vi "总磷氨氮测量流程.vi"(10 "总磷量程模式":T1, 11 "参数":T2={"站号"=1, "量程切换"=enum."AUTO", "控制命令"=enum."启动测量", "模式设置"=enum."待机", "测量间隔"=0} {"站号" items=["总磷"=1, "总氮"=2]}) -> ()   [LabVIEW 2016, in "斯坦道仪器.lvlib"]
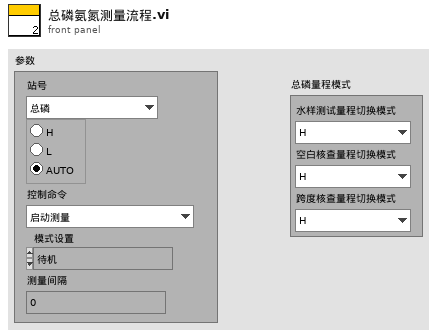
[diagram p1: front panel]
types:
  T1 = cluster{"水样测试量程切换模式":enum16{"H", "L", "AUTO"}, "空白核查量程切换模式":enum16{"H", "L", "AUTO"}, "跨度核查量程切换模式":enum16{"H", "L", "AUTO"}}
  T2 = cluster{"站号":u16, "量程切换":enum32{"H", "L", "AUTO"}, "控制命令":enum16{"启动测量", "标样核查", "零点核查", "跨度核查", "空白测试", "平行样测试", "加标回收", "空白校准", "标样校准", "初始化（清洗）", "停止测试", "仪器重启", "校时", "模式设置", "测量间隔设置"}, "模式设置":enum16{"待机", "连续模式", "周期模式", "定点模式", "受控模式", "手动模式"}, "测量间隔":u16}
  T3 = enum16{"初始化", "通电", "参数1启动", "等待参数1测试完成", "参数1测试完成", "参数1存储数据", "参数2启动", "等待参数2测试完成", "参数2测试完成", "参数2存储数据", "断电", "结束"}
  T4 = cluster{"时间标识":timestamp, "设备":string, "日志信息":string, "流程参数":string}
  T5 = cluster{"时间标识":timestamp, "监测值":sgl, "单位":u16, "数据标识":string, "因子编码":u32, "标样参考值":sgl, "F0":sgl, "F1":sgl, "F2":sgl, "F3":sgl, "F4":sgl, "F5":sgl, "F6":sgl, "F7":sgl, "X":sgl, "温度":sgl, "湿度":sgl, "量程标识":string}
  T6 = enum16{"维护数据", "水样测试", "标样核查", "零点核查", "跨度核查", "空白测试", "平行样测试", "加标回收", "空白校准", "标样校准", "初始化（清洗）"}
  T7 = enum16{"启动测量", "标样核查", "零点核查", "跨度核查", "空白测试", "平行样测试", "加标回收", "空白校准", "标样校准", "初始化（清洗）", "停止测试", "仪器重启", "校时", "模式设置", "测量间隔设置"}
  T8 = cluster{"系统时间":timestamp, "工作状态":enum16{"空闲", "水样测试", "标样核查", "零点核查", "跨度核查", "空白测试", "平行样测试", "加标回收", "空白校准", "标样校准", "初始化（清洗）"}, "测量模式":enum16{"待机", "连续模式", "周期模式", "定点模式", "受控模式", "手动模式"}, "告警代码":enum16{"无告警", "缺试剂告警", "缺水样告警", "缺蒸馏水告警", "缺标液告警", "仪表漏液告警", "标定异常告警", "超量程告警", "加热异常", "低试剂预警", "超上限告警", "超下限告警", "仪表内部其他异常", "滴定异常告警", "电极异常告警", "量程切换告警", "参数设置告警", "PH电极电位异常", "电导率电极异常", "浊度光度异常", "溶解氧电极异常", "溶解氧光强异常", "温度异常告警", "PH异常告警", "溶解氧异常告警", "电导率异常告警", "浊度异常告警", "叶绿素异常告警", "藻密度异常告警", "蓝绿藻异常告警", "ORP异常告警", "氨氮异常告警", "清洁刷异常告警", "SD卡异常告警", "蓝牙异常告警", "Wifi异常告警", "流程异常告警"}, "故障代码":enum16{"无故障", "电机故障", "温度故障", "通讯故障", "滴定故障"}, "日志代码":u16, "软件版本":u16, "F0":sgl, "F1":sgl, "F2":sgl, "F3":sgl, "T":sgl, "H":sgl, "id":u16, "flowid":u16, "量程":u16, "总磷控温温度1":sgl, "营养盐控温温度2":sgl, "ADC":sgl}
  T9 = enum16{"空闲", "水样测试", "标样核查", "零点核查", "跨度核查", "空白测试", "平行样测试", "加标回收", "空白校准", "标样校准", "初始化（清洗）"}
  T10 = cluster{"因子编码":u32, "单位":u16, "标样参考值":sgl, "水样数据时间":timestamp, "水样实测值":sgl, "水样数据标识":string, "标样数据时间":timestamp, "标样实测值":sgl, "标样数据标识":string, "空白数据时间":timestamp, "空白实测值":sgl, "空白数据标识":string, "零点核查数据时间":timestamp, "零点核查实测值":sgl, "零点核查数据标识":string, "跨度核查数据时间":timestamp, "跨度核查实测值":sgl, "跨度核查数据标识":string, "加标回收数据时间":timestamp, "加标回收实测值":sgl, "加标回收数据标识":string, "平行样数据时间":timestamp, "平行样实测值":sgl, "平行样数据标识":string, "F0":sgl, "F1":sgl, "F2":sgl, "F3":sgl, "F4":sgl, "F5":sgl, "F6":sgl, "F7":sgl, "温度":sgl, "湿度":sgl, "X值":sgl}
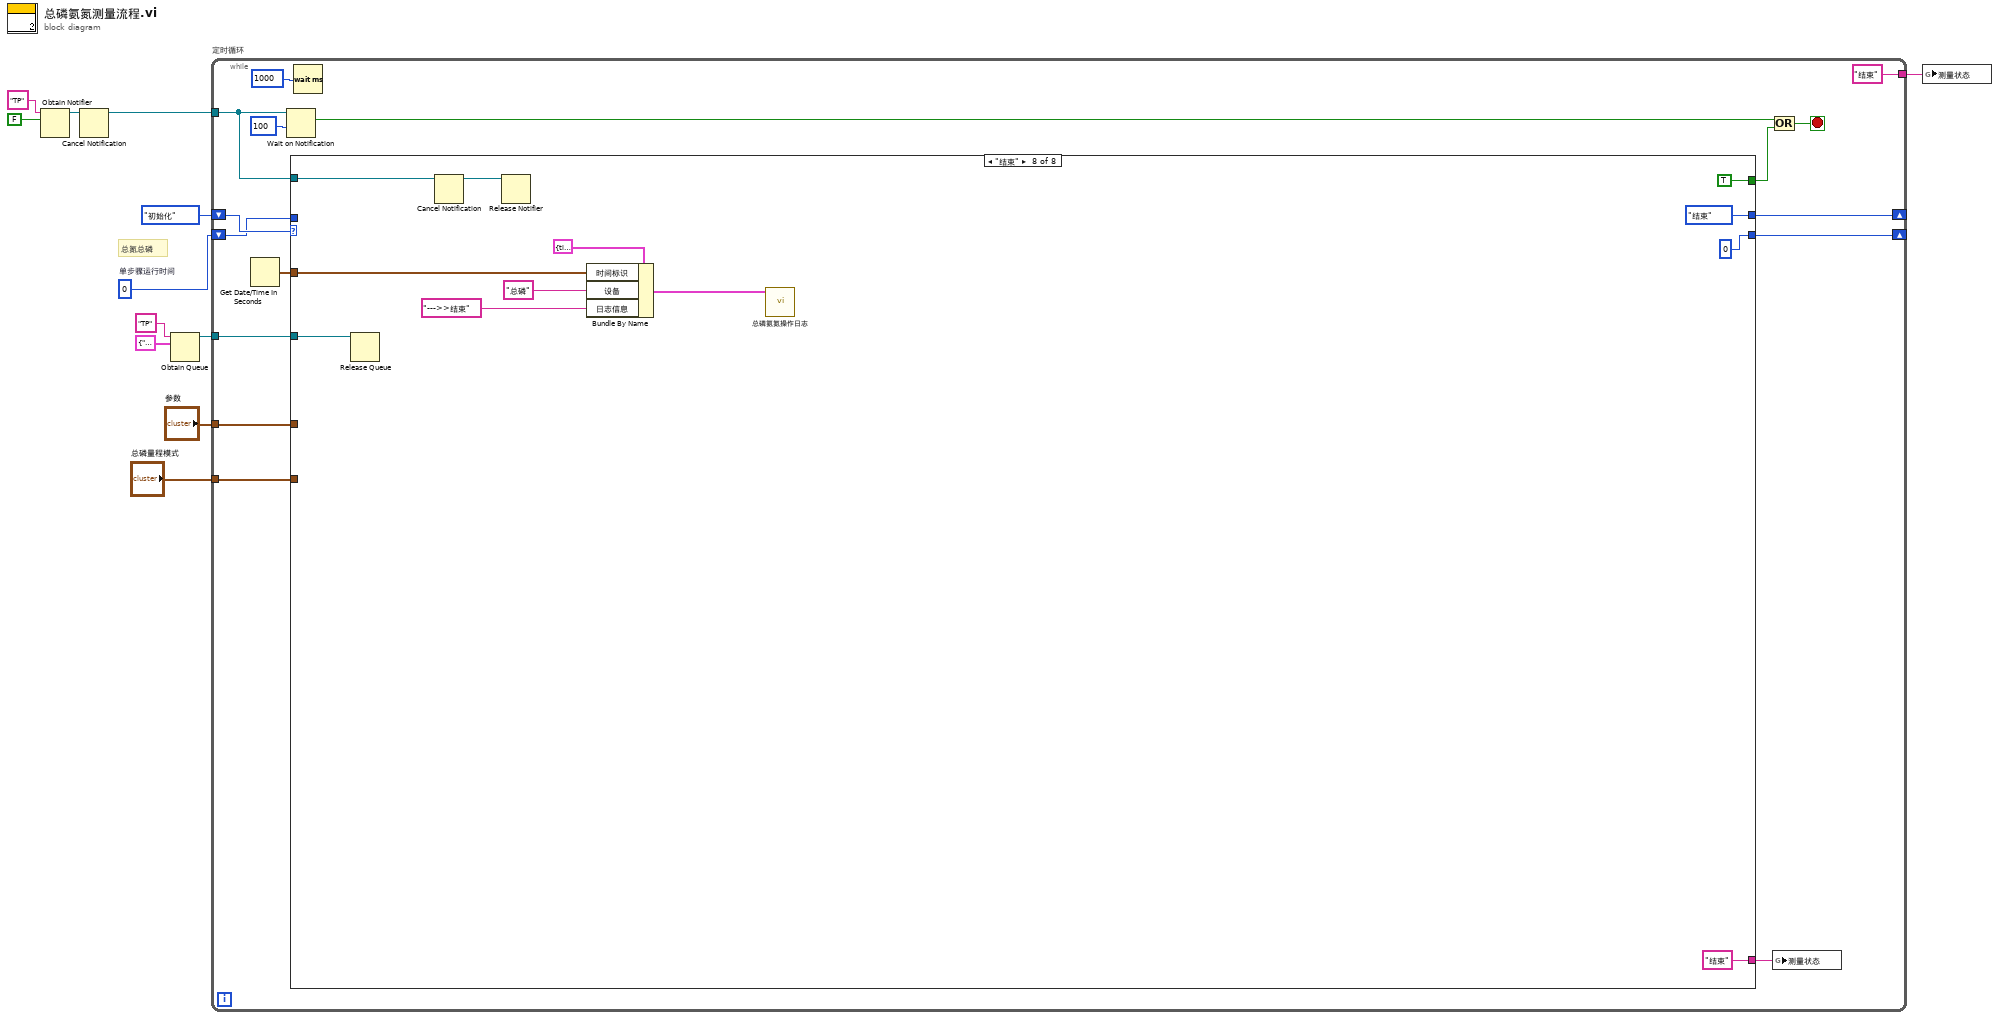
[diagram p0: block diagram]
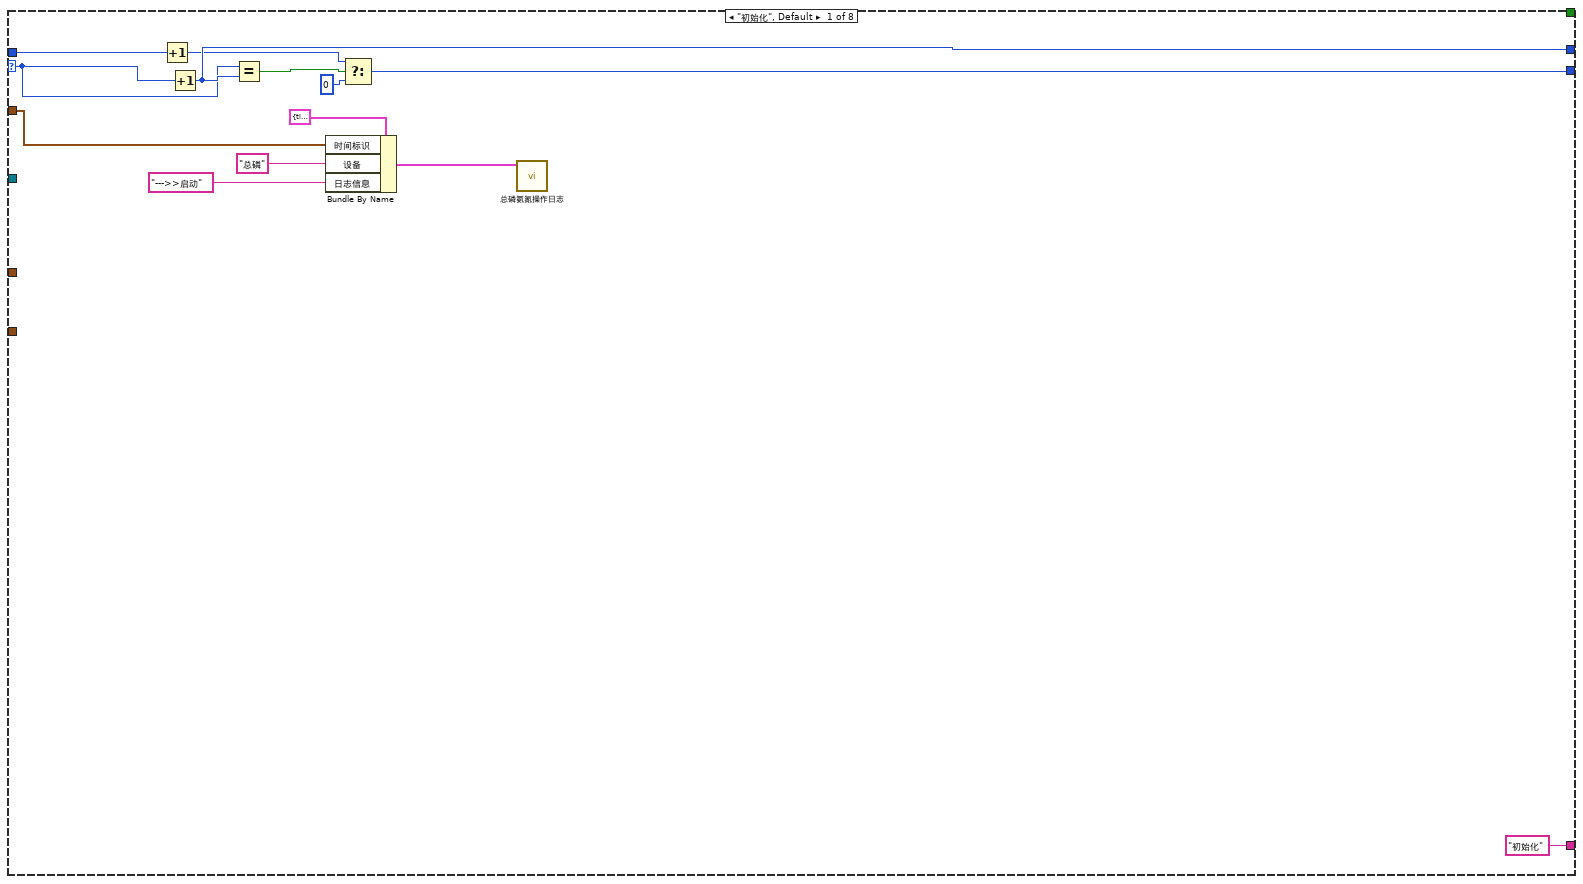
[diagram p2: hidden frame]
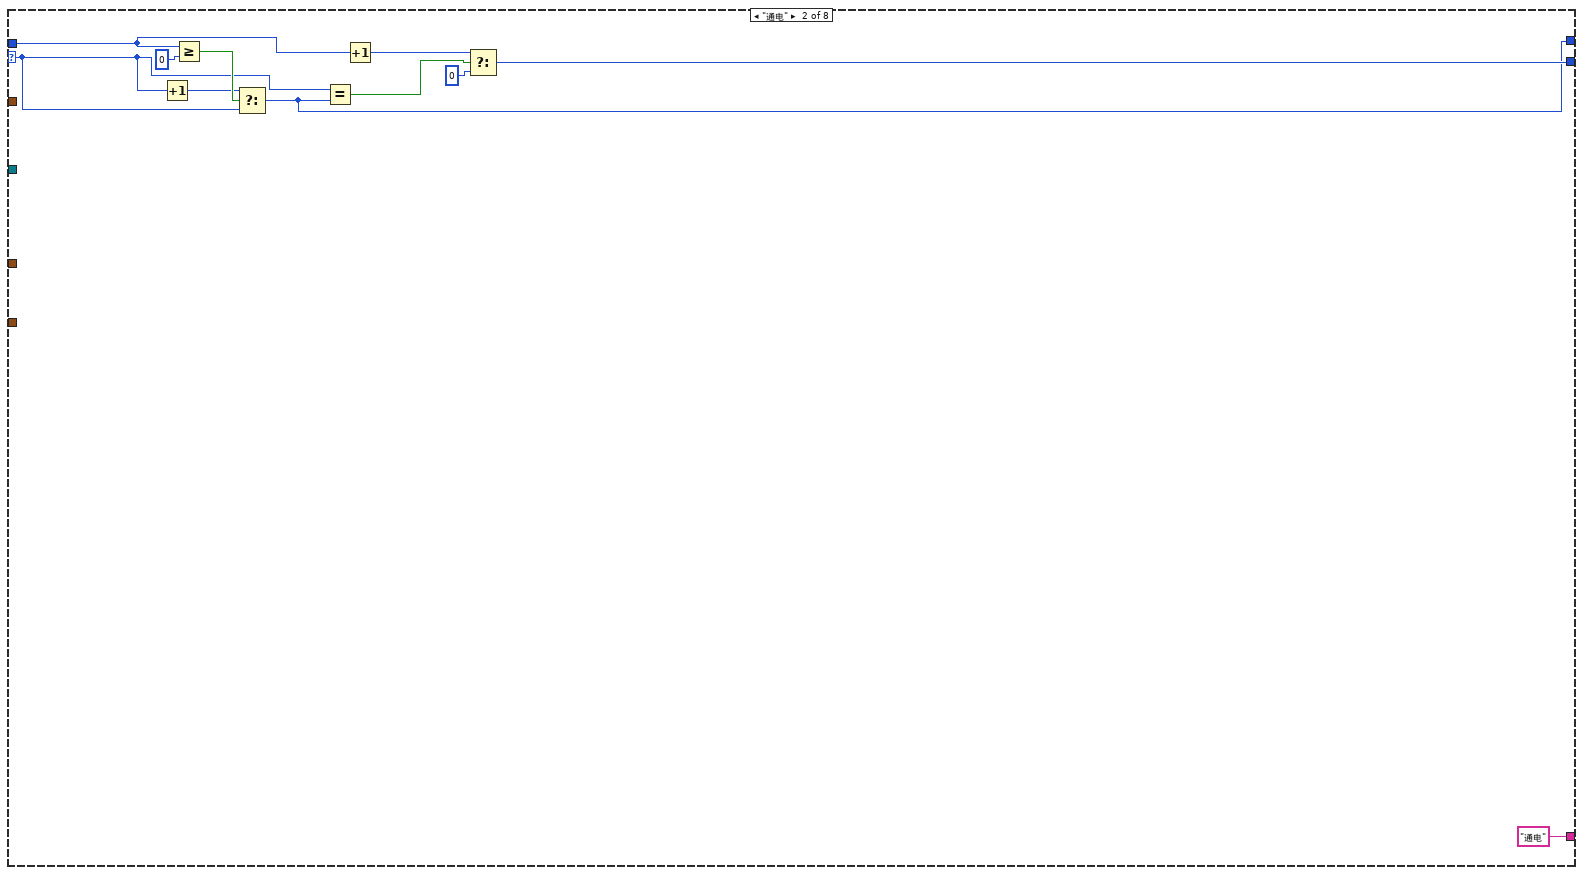
[diagram p3: hidden frame]
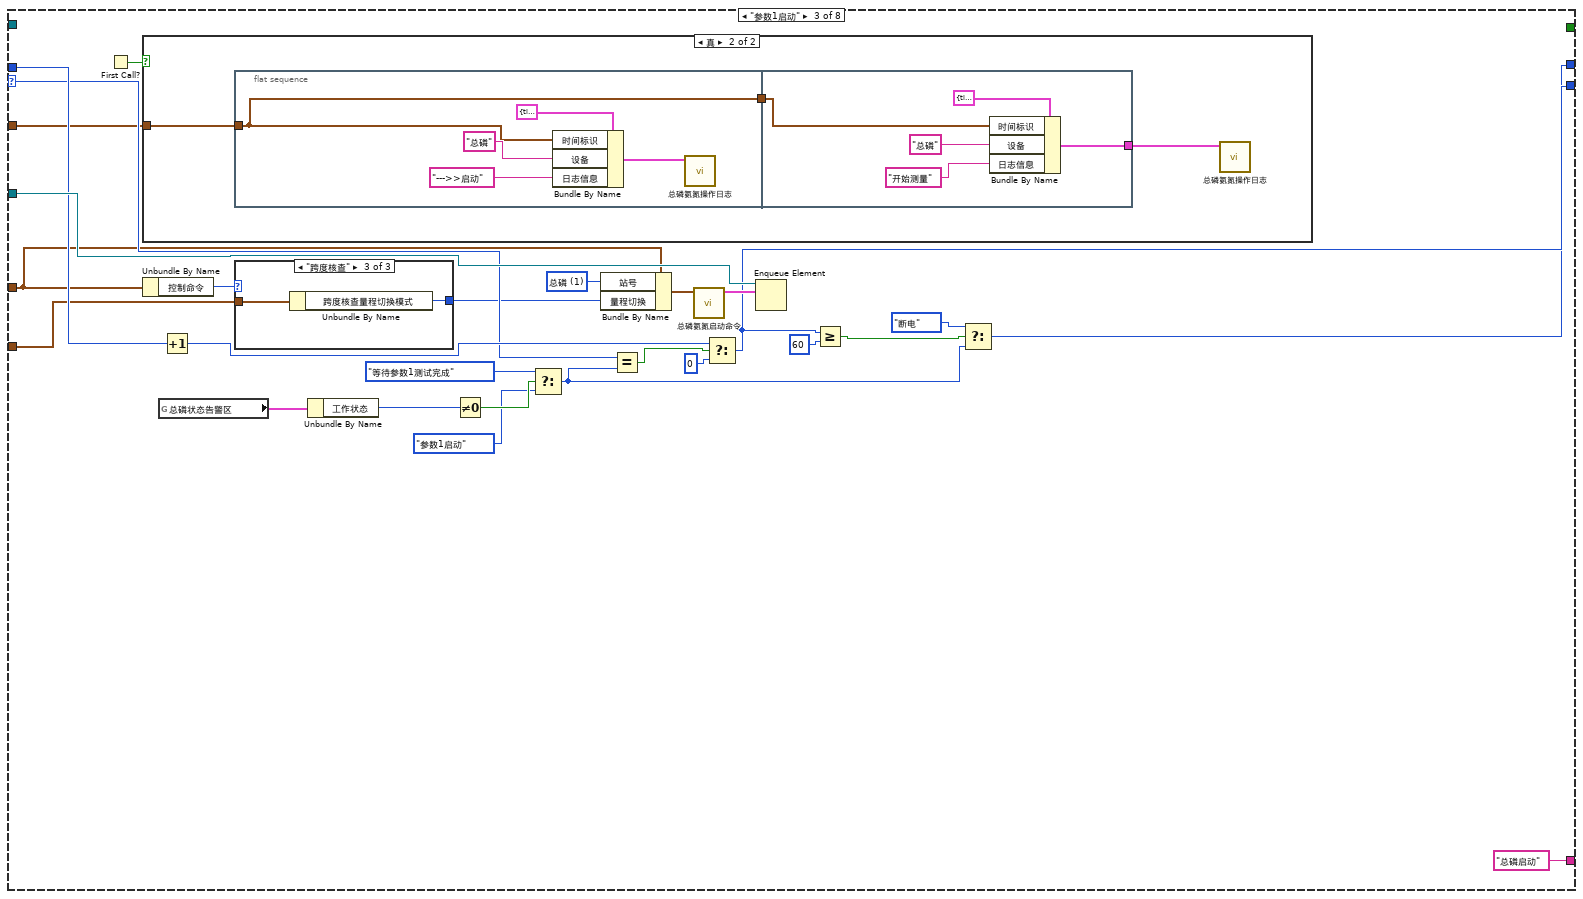
[diagram p4: hidden frame]
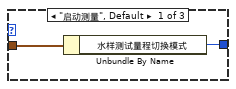
[diagram p5: hidden frame]
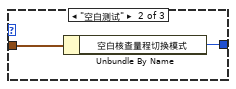
[diagram p6: hidden frame]
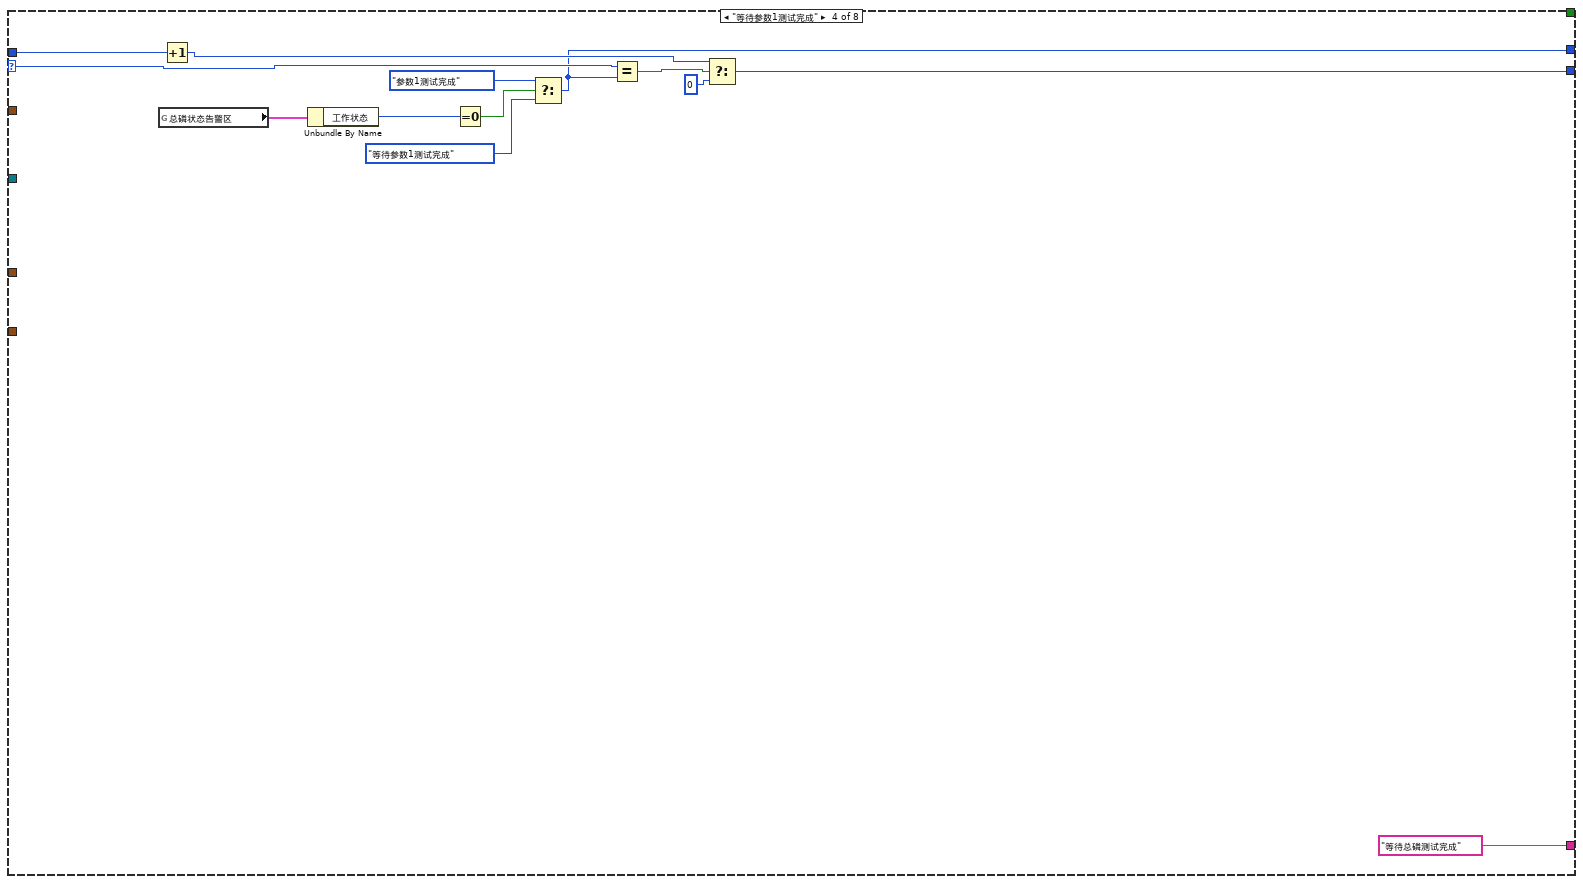
[diagram p8: hidden frame]
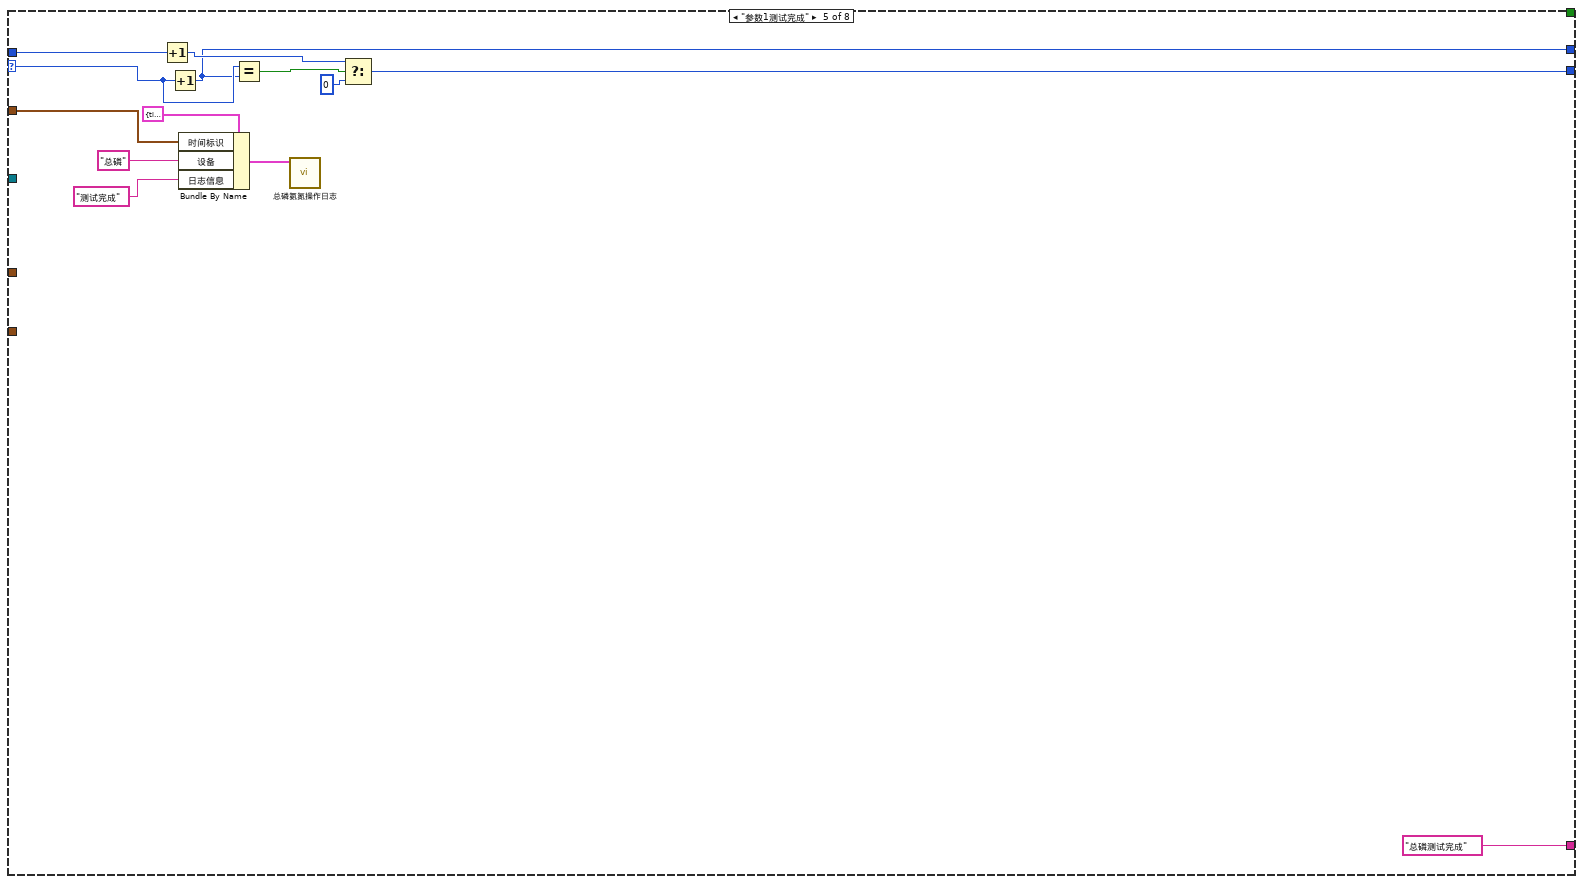
[diagram p9: hidden frame]
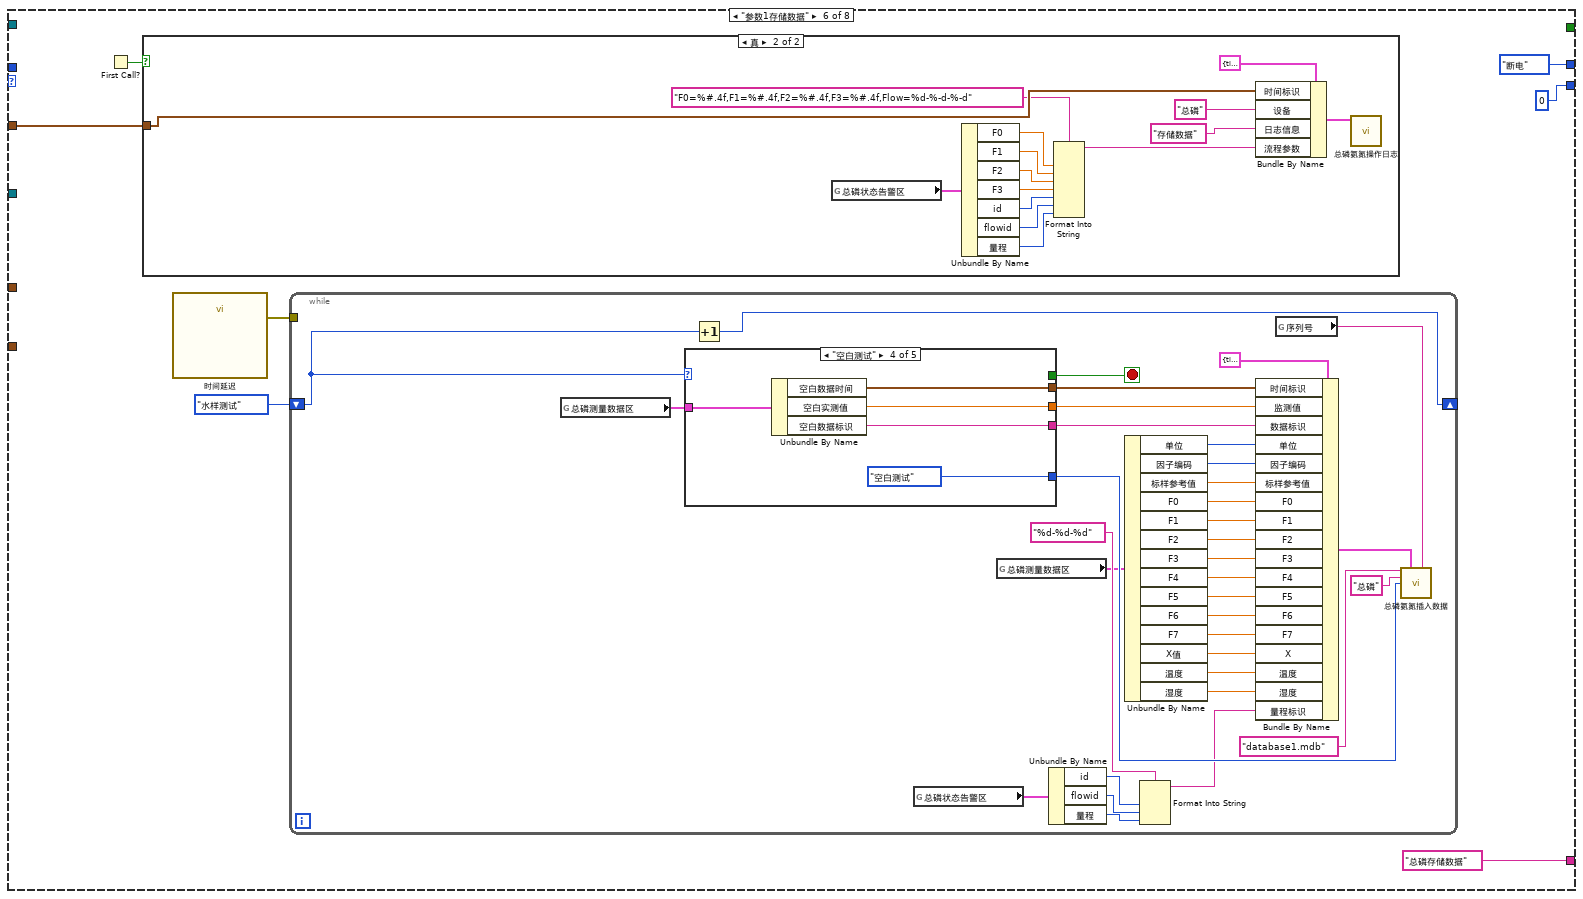
[diagram p10: hidden frame]
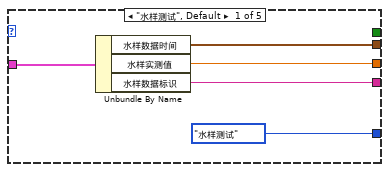
[diagram p11: hidden frame]
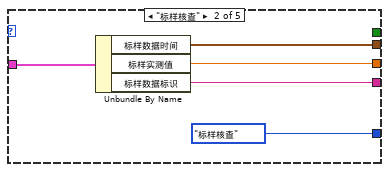
[diagram p12: hidden frame]
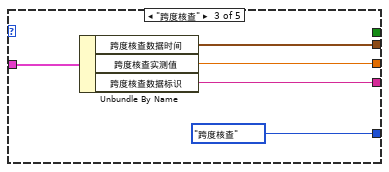
[diagram p13: hidden frame]
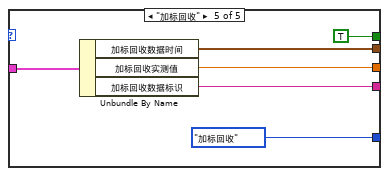
[diagram p14: hidden frame]
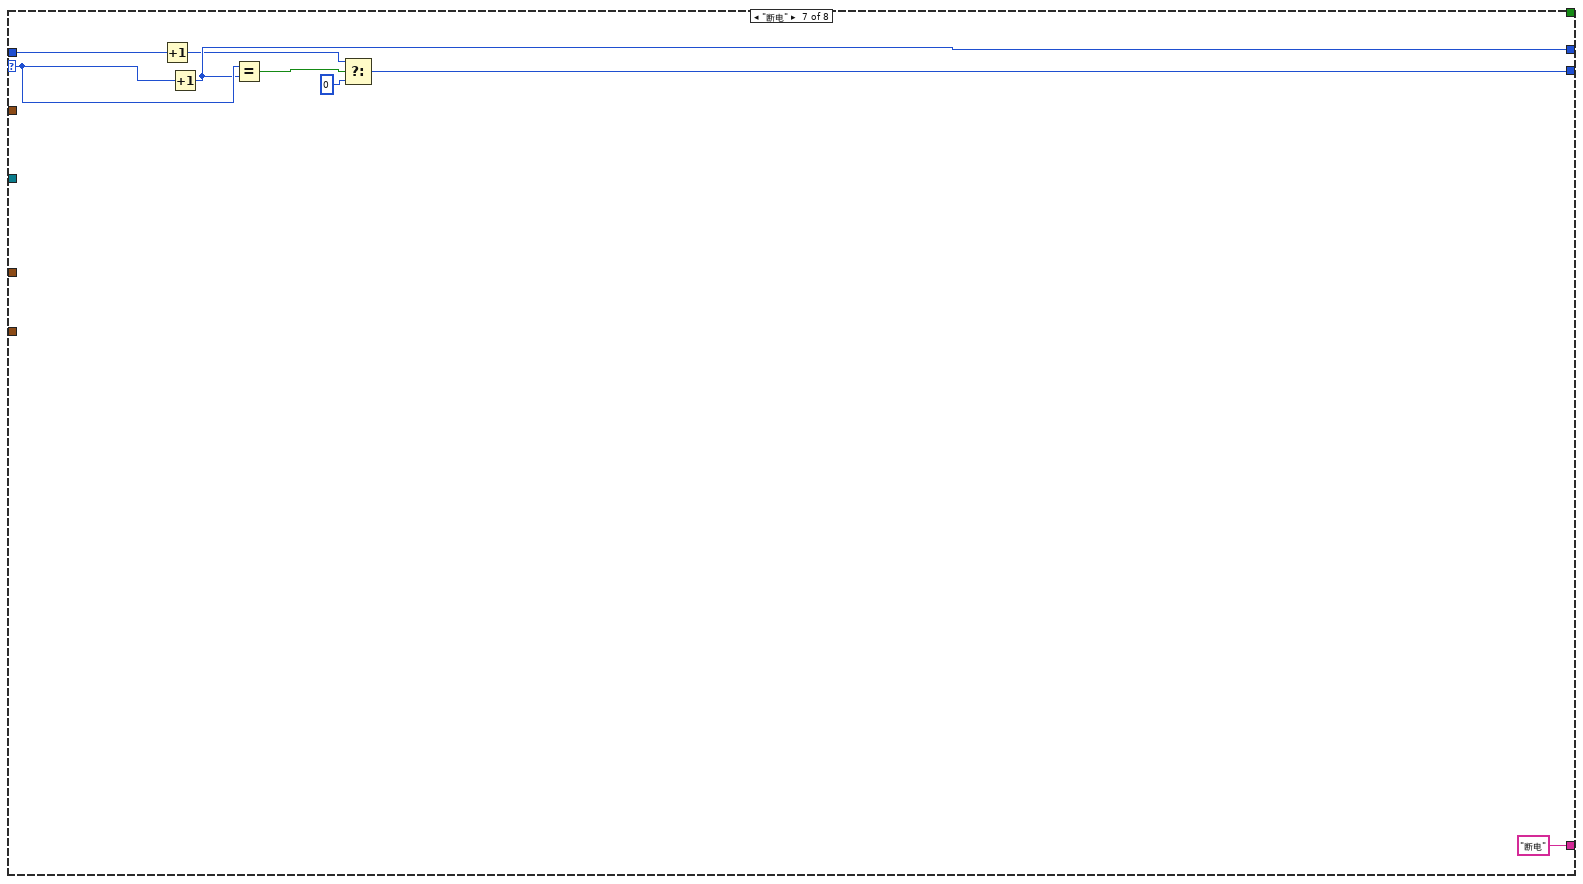
[diagram p16: hidden frame]
diagram:
  w8 = 0  # 单步骤运行时间
  # "总氮总磷"
  n1 = Obtain Notifier(name (unnamed)="TP" ("名称（未命名）"), notification data type=FALSE) -> (notifier out=w5:refnum<notifier>)  [unwired: 2 in, 2 out]
  n2 = Cancel Notification(0:w5) -> (8:w4:refnum<notifier>)  [unwired: 1 in, 2 out]
  n3 = Obtain Queue(name (unnamed)="TP" ("名称（未命名）"), element data type=cluster{"命令":string, "data":variant} {"命令"="", "data"=variant}) -> (queue out=w9:refnum<queue>)  [unwired: 3 in, 2 out]
  n4 = while "定时循环" {
    shift-right: [w27] -> _
    shift-left: T3."初始化" ("枚举") -> [w28]
    tunnel: w9 -> [w26]
    shift-right: [w24] -> _
    shift-left: w8 -> [w25]
    tunnel: w4 -> [w23]
    tunnel: "参数" -> [w18]
    tunnel: "总磷量程模式" -> [w15]
    tunnel: ["结束" ("输入 1")] -> w1
    stop <- w19 stop-if-true
    n5 = Get Date/Time In Seconds() -> (seconds since 1Jan1904=w16:timestamp)
    n6 = Wait on Notification(notifier=w23, timeout in ms (-1)=100 ("超时毫秒(-1)")) -> (notification=w20:bool)  [unwired: 2 in, 3 out]
    n7 = case shown="\"结束\"" w28 {
      selector: w28 -> [w39 w46 w68 w104 w120 _ w212 _]
      tunnel: [_ _ _ _ _ _ _ TRUE] -> w21
      tunnel: [w40 w45 w53 w102 w118 T3."断电" ("枚举") w211 T3."结束" ("枚举")] -> w27
      tunnel: w26 -> [_ _ w76 _ _ _ _ w224]
      tunnel: w25 -> [w41 w47 w69 w105 w121 _ w214 _]
      tunnel: [w37 w48 w54 w103 w119 0 ("t") w213 0 ("t")] -> w24
      tunnel: w23 -> [_ _ _ _ _ _ _ w223]
      tunnel: w18 -> [_ _ w62 _ _ _ _ _]
      tunnel: w16 -> [w30 _ w67 _ w113 w130 _ w217]
      tunnel: ["初始化" ("输入 1") "通电" ("输入 1") "总磷启动" ("输入 1") "等待总磷测试完成" ("输入 1") "总磷测试完成" ("输入 1") "总磷存储数据" ("输入 1") "断电" ("输入 1") "结束" ("输入 1")] -> w14
      tunnel: w15 -> [_ _ w60 _ _ _ _ _]
      frame "初始化", Default {
        n8 = Increment(x=w41) -> (x+1=w35:i32)
        n9 = Increment(x=w39) -> (x+1=w40:T3)
        n10 = Equal?(x=w39, y=w40) -> (x = y?=w38:bool)
        n11 = Bundle By Name(cluster=T4 {"时间标识"=timestamp(0 s since 1904-01-01), "设备"="", "日志信息"="", "流程参数"=""} ("data in"), "时间标识"=w30, "设备"="总磷", "日志信息"="--->>启动") -> (w34:T4)
        n12 = Select(t=w35, s=w38, f=0 ("t")) -> (s? t:f=w37:i32)
        n13 = call "总磷氨氮操作日志.vi"("data in"=w34) -> ()  [unwired: 11 in]
      }
      frame "通电" {
        n14 = Increment(x=w46) -> (x+1=w50:T3)
        n15 = Greater Or Equal?(x=w47, y=0) -> (x >= y?=w51:bool)
        n16 = Select(t=w50, s=w51, f=w46) -> (s? t:f=w45:T3)
        n17 = Equal?(x=w46, y=w45) -> (x = y?=w49:bool)
        n18 = Increment(x=w47) -> (x+1=w44:i32)
        n19 = Select(t=w44, s=w49, f=0 ("t")) -> (s? t:f=w48:i32)
      }
      frame "参数1启动" {
        w77 = u16 1 items=["总氮"=2, "总磷"=1] ("站号")
        n20 = First Call?() -> (First Call?: T/F=w66:bool)
        n21 = case shown="真" w66 {
          tunnel: w67 -> [_ w86]
          frame False {
          }
          frame True {
            n22 = flat-sequence {
              tunnel: w86 -> [w89]
              tunnel: [w89] -> w87
              tunnel: [w98] -> w88
              tunnel: w87 -> [w94]
              frame #0 {
                n23 = Bundle By Name(cluster=T4 {"时间标识"=timestamp(0 s since 1904-01-01), "设备"="", "日志信息"="", "流程参数"=""} ("data in"), "时间标识"=w89, "设备"="总磷", "日志信息"="--->>启动") -> (w93:T4)
                n24 = call "总磷氨氮操作日志.vi"("data in"=w93) -> ()  [unwired: 11 in]
              }
              frame #1 {
                n25 = Bundle By Name(cluster=T4 {"时间标识"=timestamp(0 s since 1904-01-01), "设备"="", "日志信息"="", "流程参数"=""} ("data in"), "时间标识"=w94, "设备"="总磷", "日志信息"="开始测量") -> (w98:T4)
              }
            }
            n26 = call "总磷氨氮操作日志.vi"("data in"=w88) -> ()  [unwired: 11 in]
          }
        }
        n27 = Unbundle By Name(w62) -> ("控制命令"=w61:T7)
        n28 = global read "VAR总磷氨氮全局变量.vi" "总磷状态告警区"() -> (w70:T8)
        n29 = Increment(x=w69) -> (x+1=w71:i32)
        n30 = case shown="\"跨度核查\"" w61 {
          tunnel: w60 -> [w81 w83 w85]
          tunnel: [w80 w82 w84] -> w59
          frame "启动测量", Default {
            n31 = Unbundle By Name(w81) -> ("水样测试量程切换模式"=w80:enum16{"H", "L", "AUTO"})
          }
          frame "空白测试" {
            n32 = Unbundle By Name(w83) -> ("空白核查量程切换模式"=w82:enum16{"H", "L", "AUTO"})
          }
          frame "跨度核查" {
            n33 = Unbundle By Name(w85) -> ("跨度核查量程切换模式"=w84:enum16{"H", "L", "AUTO"})
          }
        }
        n34 = Unbundle By Name(w70) -> ("工作状态"=w75:T9)
        n35 = Not Equal To 0?(x=w75) -> (x != 0?=w74:bool)
        n36 = Select(t=T3."等待参数1测试完成" ("枚举"), s=w74, f=T3."参数1启动" ("枚举")) -> (s? t:f=w55:T3)
        n37 = Bundle By Name(cluster=w62, "站号"=w77, "量程切换"=w59) -> (w78:T2)
        n38 = Equal?(x=w68, y=w55) -> (x = y?=w73:bool)
        n39 = call "总磷氨氮启动命令.vi"("参数"=w78) -> ("启动命令"=w79:cluster{"命令":string, "data":variant})  [unwired: 10 in]
        n40 = Select(t=w71, s=w73, f=0 ("t")) -> (s? t:f=w54:i32)
        n41 = Enqueue Element(queue=w76, element=w79) -> ()  [unwired: 2 in, 3 out]
        n42 = Greater Or Equal?(x=w54, y=60) -> (x >= y?=w57:bool)
        n43 = Select(t=T3."断电" ("枚举"), s=w57, f=w55) -> (s? t:f=w53:T3)
      }
      frame "等待参数1测试完成" {
        n44 = global read "VAR总磷氨氮全局变量.vi" "总磷状态告警区"() -> (w106:T8)
        n45 = Increment(x=w105) -> (x+1=w107:i32)
        n46 = Unbundle By Name(w106) -> ("工作状态"=w111:T9)
        n47 = Equal To 0?(x=w111) -> (x = 0?=w110:bool)
        n48 = Select(t=T3."参数1测试完成" ("枚举"), s=w110, f=T3."等待参数1测试完成" ("枚举")) -> (s? t:f=w102:T3)
        n49 = Equal?(x=w104, y=w102) -> (x = y?=w109:bool)
        n50 = Select(t=w107, s=w109, f=0 ("t")) -> (s? t:f=w103:i32)
      }
      frame "参数1测试完成" {
        n51 = Increment(x=w121) -> (x+1=w122:i32)
        n52 = Increment(x=w120) -> (x+1=w118:T3)
        n53 = Bundle By Name(cluster=T4 {"时间标识"=timestamp(0 s since 1904-01-01), "设备"="", "日志信息"="", "流程参数"=""} ("data in"), "时间标识"=w113, "设备"="总磷", "日志信息"="测试完成") -> (w117:T4)
        n54 = Equal?(x=w120, y=w118) -> (x = y?=w124:bool)
        n55 = call "总磷氨氮操作日志.vi"("data in"=w117) -> ()  [unwired: 11 in]
        n56 = Select(t=w122, s=w124, f=0 ("t")) -> (s? t:f=w119:i32)
      }
      frame "参数1存储数据" {
        n57 = First Call?() -> (First Call?: T/F=w127:bool)
        n58 = case shown="真" w127 {
          tunnel: w130 -> [_ w202]
          frame False {
          }
          frame True {
            n59 = global read "VAR总磷氨氮全局变量.vi" "总磷状态告警区"() -> (w201:T8)
            n60 = Unbundle By Name(w201) -> ("F0"=w193:sgl, "F1"=w194:sgl, "F2"=w195:sgl, "F3"=w196:sgl, "id"=w197:u16, "flowid"=w198:u16, "量程"=w199:u16)
            n61 = Format Into String(format string="F0=%#.4f,F1=%#.4f,F2=%#.4f,F3=%#.4f,Flow=%d-%-d-%-d" ("格式字符串"), w193, w194, w195, w196, w197, w198, w199) -> (resulting string=w192:string)  [unwired: 2 in, 1 out]
            n62 = Bundle By Name(cluster=T4 {"时间标识"=timestamp(0 s since 1904-01-01), "设备"="", "日志信息"="", "流程参数"=""} ("data in"), "时间标识"=w202, "设备"="总磷", "日志信息"="存储数据", "流程参数"=w192) -> (w206:T4)
            n63 = call "总磷氨氮操作日志.vi"("data in"=w206) -> ()  [unwired: 11 in]
          }
        }
        n64 = call "时间延迟"() -> ("error out"=w125:errorcluster)  [unwired: 11 in]
        n65 = while {
          shift-right: [w148] -> _
          shift-left: enum16{"水样测试", "标样核查", "跨度核查", "空白测试", "加标回收"}."水样测试" ("测量模式") -> [w149]
          tunnel: w125 -> [_]
          stop <- w150 stop-if-true
          n66 = global read "VAR总磷氨氮全局变量.vi" "总磷测量数据区"() -> (w147:T10)
          n67 = case shown="\"空白测试\"" w149 {
            tunnel: w147 -> [w170 w175 w180 w185 w191]
            tunnel: [w169 w174 w179 w184 w190] -> w154
            tunnel: [w168 w173 w178 w183 w189] -> w153
            tunnel: [w167 w172 w177 w182 w188] -> w152
            tunnel: [T6."水样测试" ("测量模式") T6."标样核查" ("测量模式") T6."跨度核查" ("测量模式") T6."空白测试" ("测量模式") T6."加标回收" ("测量模式")] -> w151
            tunnel: [_ _ _ _ TRUE] -> w150
            frame "水样测试", Default {
              n68 = Unbundle By Name(w170) -> ("水样数据时间"=w169:timestamp, "水样实测值"=w168:sgl, "水样数据标识"=w167:string)
            }
            frame "标样核查" {
              n69 = Unbundle By Name(w175) -> ("标样数据时间"=w174:timestamp, "标样实测值"=w173:sgl, "标样数据标识"=w172:string)
            }
            frame "跨度核查" {
              n70 = Unbundle By Name(w180) -> ("跨度核查数据时间"=w179:timestamp, "跨度核查实测值"=w178:sgl, "跨度核查数据标识"=w177:string)
            }
            frame "空白测试" {
              n71 = Unbundle By Name(w185) -> ("空白数据时间"=w184:timestamp, "空白实测值"=w183:sgl, "空白数据标识"=w182:string)
            }
            frame "加标回收" {
              n72 = Unbundle By Name(w191) -> ("加标回收数据时间"=w190:timestamp, "加标回收实测值"=w189:sgl, "加标回收数据标识"=w188:string)
            }
          }
          n73 = Increment(x=w149) -> (x+1=w148:enum16{"水样测试", "标样核查", "跨度核查", "空白测试", "加标回收"})
          n74 = global read "VAR总磷氨氮全局变量.vi" "总磷状态告警区"() -> (w162:T8)
          n75 = global read "VAR总磷氨氮全局变量.vi" "总磷测量数据区"() -> (w146:T10)
          n76 = Unbundle By Name(w162) -> ("id"=w158:u16, "flowid"=w157:u16, "量程"=w156:u16)
          n77 = Unbundle By Name(w146) -> ("单位"=w165:u16, "因子编码"=w164:u32, "标样参考值"=w163:sgl, "F0"=w132:sgl, "F1"=w133:sgl, "F2"=w134:sgl, "F3"=w135:sgl, "F4"=w136:sgl, "F5"=w137:sgl, "F6"=w138:sgl, "F7"=w139:sgl, "X值"=w140:sgl, "温度"=w141:sgl, "湿度"=w142:sgl)
          n78 = Format Into String(format string="%d-%d-%d" ("格式字符串"), w158, w157, w156) -> (resulting string=w143:string)  [unwired: 2 in, 1 out]
          n79 = Bundle By Name(cluster=T5 {"时间标识"=timestamp(0 s since 1904-01-01), "监测值"=0.0, "单位"=0, "数据标识"="", "因子编码"=0, "标样参考值"=0.0, "F0"=0.0, "F1"=0.0, "F2"=0.0, "F3"=0.0, "F4"=0.0, "F5"=0.0, "F6"=0.0, "F7"=0.0, "X"=0.0, "温度"=0.0, "湿度"=0.0, "量程标识"=""} ("data"), "时间标识"=w154, "监测值"=w153, "数据标识"=w152, "单位"=w165, "因子编码"=w164, "标样参考值"=w163, "F0"=w132, "F1"=w133, "F2"=w134, "F3"=w135, "F4"=w136, "F5"=w137, "F6"=w138, "F7"=w139, "X"=w140, "温度"=w141, "湿度"=w142, "量程标识"=w143) -> (w145:T5)
          n80 = global read "VAR总磷氨氮全局变量.vi" "序列号"() -> (w155:string)
          n81 = call "总磷氨氮插入数据.vi"("database"="database1.mdb", "data"=w145, "SN"=w155, "table"="总磷", "测量模式"=w151) -> ()  [unwired: 10 in, 1 out]
        }
      }
      frame "断电" {
        n82 = Increment(x=w214) -> (x+1=w207:i32)
        n83 = Increment(x=w212) -> (x+1=w211:T3)
        n84 = Equal?(x=w212, y=w211) -> (x = y?=w209:bool)
        n85 = Select(t=w207, s=w209, f=0 ("t")) -> (s? t:f=w213:i32)
      }
      frame "结束" {
        n86 = Release Queue(queue=w224) -> ()  [unwired: 2 in, 3 out]
        n87 = Cancel Notification(0:w223) -> (8:w222:refnum<notifier>)  [unwired: 1 in, 2 out]
        n88 = Release Notifier(notifier=w222) -> ()  [unwired: 2 in, 3 out]
        n89 = Bundle By Name(cluster=T4 {"时间标识"=timestamp(0 s since 1904-01-01), "设备"="", "日志信息"="", "流程参数"=""} ("data in"), "时间标识"=w217, "设备"="总磷", "日志信息"="--->>结束") -> (w221:T4)
        n90 = call "总磷氨氮操作日志.vi"("data in"=w221) -> ()  [unwired: 11 in]
      }
    }
    n91 = Wait (ms)(milliseconds to wait=u32 1000 ("等待时间（毫秒）")) -> ()  [unwired: 1 out]
    n92 = Or(x=w20, y=w21) -> (x .or. y?=w19:bool)
    n93 = global write "VAR总磷氨氮全局变量.vi" "测量状态"(w14) -> ()
  }
  n94 = global write "VAR总磷氨氮全局变量.vi" "测量状态"(w1) -> ()
